vi "Grava_conditionsACQ.vi"(0 "ACQ Parameters (cluster)":T2={"Acquisition Mode"=0, "Pulse width"=0, "DTP period"=3, "Number of events"=100000} caption="Acquisition Parameters" {"Number of events" min=1 max=166666; "DTP period" min=1; "Pulse width" items=["25 ns", "50 ns", "75 ns", "100 ns"]; "Acquisition Mode" items=["Normal", "Pedestal", "Test Pulse", "Test Pulse trigger & synchronous"]}, 1 "HV parameters":T1={"Final value"=-300, "Number of steps"=10, "Time/step"=800, "Output Off Behavior"=0, "VISA resource name"="GPIB1::25::INSTR"} {"Output Off Behavior" items=["Normal", "High Impedance", "Zero", "Guard"]; "Time/step" min=100 max=2000 step=100; "Final value" min=-1100 max=0 step=10; "Number of steps" min=10 max=20 step=10}, 2 "ACQ events fets":u32 caption="Acquired events" format="%#.8p", 3 "EQ folder path":string, 4 "ACQ folder path":path, 5 "EQ loaded?":bool, 6 "etapa2 Waiting time (s)":u32=50 caption="Waiting time\nbefore operation (s)" min=1, 7 "ACQ anVref low":u8(ring)=32 caption="Analog Vref low (V)" items=["0.4", "0.415625", "0.43125", "0.446875", "0.4625", "0.478125", "0.49375", "0.509375", "0.525", "0.540625", "0.55625", "0.571875", "0.5875", "0.603125", "0.61875", "0.634375", "0.65", "0.665625", "0.68125", "0.696875", "0.7125", "0.728125", "0.74375", "0.759375", "0.775", "0.790625", "0.80625", "0.821875", "0.8375", "0.853125", "0.86875", "0.884375", "0.9", "0.915625", "0.93125", "0.946875", "0.9625", "0.978125", "0.99375", "1.009375", "1.025", "1.040625", "1.05625", "1.071875", "1.0875", "1.103125", "1.11875", "1.134375", "1.15", "1.165625", "1.18125", "1.196875", "1.2125", "1.228125", "1.24375", "1.259375", "1.275", "1.290625", "1.30625", "1.321875", "1.3375", "1.353125", "1.36875", "1.384375"], 8 "Acquisition time (s)":u32=180 min=1, 9 "ACQ GbTHLD":u8(ring)=22 caption="Global threshold (V)" items=["0.34", "0.37", "0.40", "0.43", "0.45", "0.48", "0.51", "0.54", "0.57", "0.60", "0.63", "0.65", "0.68", "0.71", "0.74", "0.77", "0.80", "0.82", "0.85", "0.88", "0.91", "0.94", "0.97", "0.99", "1.02", "1.05", "1.08", "1.11", "1.14", "1.16", "1.19", "1.22", "1.25", "1.28", "1.31", "1.34", "1.36", "1.39", "1.42", "1.45", "1.48", "1.51", "1.53", "1.56", "1.59", "1.62", "1.65", "1.68", "1.70", "1.73", "1.76", "1.79", "1.82", "1.85", "1.88", "1.90", "1.93", "1.96", "1.99", "2.02", "2.05", "2.07", "2.10", "2.13"], 10 "etapa5 Waiting time (s)":u32=120 caption="Waiting time\nfor next iteration (s)" min=1, 11 "HV loops":i32, 13 "Total ACQ time (s)":u32) -> ()   [LabVIEW 2015, in "VIPM2.lvlib"]
uses:
  VIPM2.lvlib
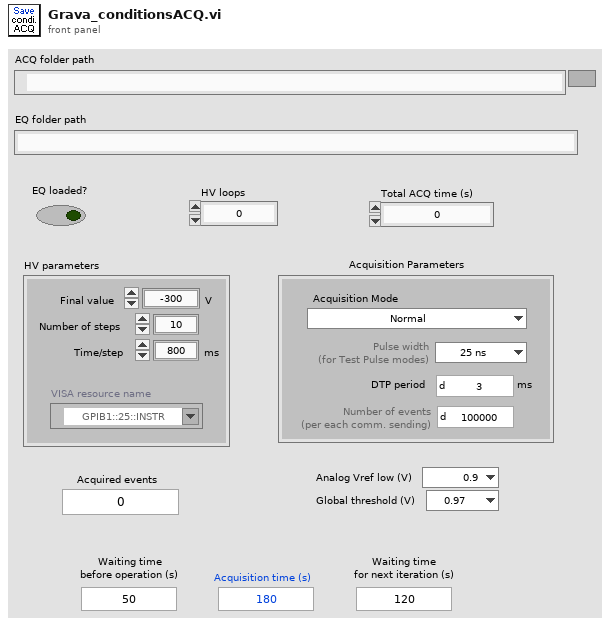
[diagram p1: front panel]
types:
  T1 = cluster{"Final value":i16, "Number of steps":u8, "Time/step":u16, "Output Off Behavior":u16, "VISA resource name":refnum<visa-resource-name>}
  T2 = cluster{"Acquisition Mode":u32, "Pulse width":u32, "DTP period":u32, "Number of events":u32}
  T3 = enum16{"open", "replace", "create", "open or create", "replace or create", "replace or create with confirmation"}
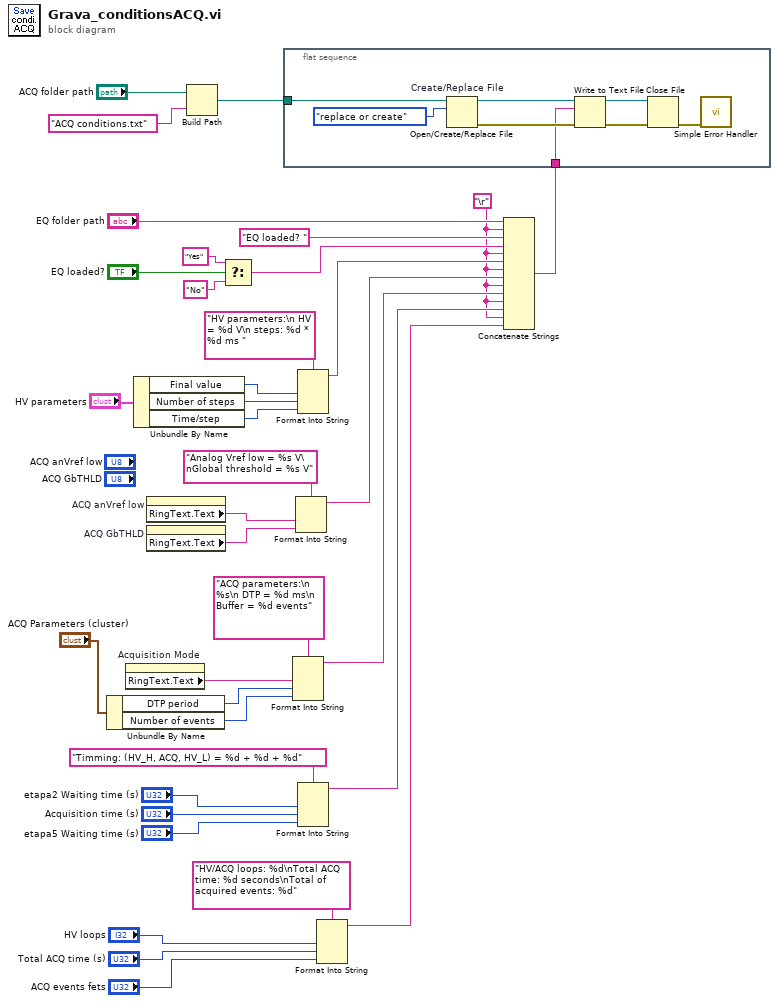
[diagram p0: block diagram]
diagram:
  w3 = "\r"
  n1 = Unbundle By Name("ACQ Parameters (cluster)") -> ("DTP period"=w11:u32, "Number of events"=w10:u32)
  n2 = property on="Acquisition Mode" class="Ring (strict)"() -> ("RingText.Text"=w12:string)  [unwired: 2 in, 2 out]
  n3 = Unbundle By Name("HV parameters") -> ("Final value"=w21:i16, "Number of steps"=w22:u8, "Time/step"=w20:u16)
  n4 = property on="ACQ anVref low" class="Ring (strict)"() -> ("RingText.Text"=w17:string)  [unwired: 2 in, 2 out]
  n5 = property on="ACQ GbTHLD" class="Ring (strict)"() -> ("RingText.Text"=w16:string)  [unwired: 2 in, 2 out]
  n6 = Build Path(base path="ACQ folder path", name or relative path="ACQ conditions.txt") -> (appended path=w35:path)
  n7 = Select(t="Yes", s="EQ loaded?", f="No") -> (s? t:f=w29:string)
  n8 = flat-sequence {
    tunnel: w35 -> [w45]
    tunnel: w25 -> [w38]
    frame #0 {
      n9 = Open/Create/Replace File "Create/Replace File"(file path (use dialog)=w45, operation (0:open)=T3."replace or create") -> (refnum out=w43:refnum<file>, error out=w42:errorcluster)  [unwired: 4 in, 1 out]
      n10 = Write to Text File(file (use dialog)=w43, text=w38, error in=w42) -> (refnum out=w41:refnum<file>, error out=w40:errorcluster)  [unwired: 1 in, 1 out]
      n11 = Close File(refnum=w41, error in=w40) -> (error out=w39:errorcluster)  [unwired: 1 out]
      n12 = call <vilib>:"Simple Error Handler.vi"("error in (no error)"=w39) -> ()  [unwired: 4 in, 5 out]
    }
  }
  n13 = Format Into String "Format Into String"(format string="ACQ parameters:\n %s\n DTP = %d ms\n Buffer = %d events", w12, w11, w10) -> (resulting string=w9:string)  [unwired: 2 in, 1 out]
  n14 = Format Into String "Format Into String"(format string="Analog Vref low = %s V\nGlobal threshold = %s V", w17, w16) -> (resulting string=w15:string)  [unwired: 2 in, 1 out]
  n15 = Format Into String "Format Into String"(format string="HV parameters:\n HV = %d V\n steps: %d * %d ms ", w21, w22, w20) -> (resulting string=w19:string)  [unwired: 2 in, 1 out]
  n16 = Format Into String "Format Into String"(format string="Timming: (HV_H, ACQ, HV_L) = %d + %d + %d", "etapa2 Waiting time (s)", "Acquisition time (s)", "etapa5 Waiting time (s)") -> (resulting string=w4:string)  [unwired: 2 in, 1 out]
  n17 = Format Into String "Format Into String"(format string="HV/ACQ loops: %d\nTotal ACQ time: %d seconds\nTotal of acquired events: %d", "HV loops", "Total ACQ time (s)", "ACQ events fets") -> (resulting string=w1:string)  [unwired: 2 in, 1 out]
  n18 = Concatenate Strings "Concatenate Strings"("EQ folder path", w3, "EQ loaded? ", w29, w3, w19, w3, w15, w3, w9, w3, w4, w3, w1) -> (w25:string)
